vi "Convert filetype to Is VI.vi"(4 "file type":T1) -> (1 "Is VI?":bool)   [LabVIEW 2019, in "NI_FileType.lvlib"]
doc: "Returns TRUE if this file type could be loaded with the Open VI Reference function. It includes VIs, Polymorphic VIs, Controls, Templates, and Globals."
uses:
  NI_FileType.lvlib
  FT_FileTypes.ctl
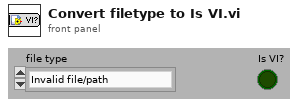
[diagram p1: front panel]
types:
  T1 = typedef "NI_FileType.lvlib/FT_FileTypes.ctl" = enum32{"Invalid file/path", "Unknown type", "Instrument", "Control", "Polymorphic VI", "Project", "Library", "LVClass", "XControl", "XNode", "CIN", "Run-time menu", "Palette menu", "LLB", "Shortcut", "Directory", "Class Private Data Control", "Statechart", "MathScript .m file", "Ladder Diagram", "LVLibp"}
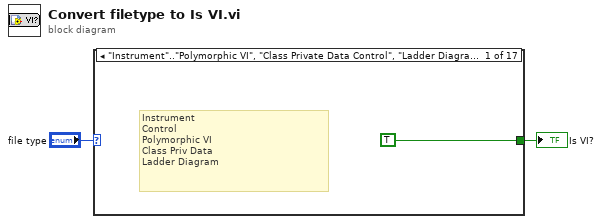
[diagram p0: block diagram]
diagram:
  n1 = case shown="\"Instrument\"..\"Polymorphic VI\", \"Class Private Data Control\", \"Ladder Diagram\"" "file type" {
    tunnel: [TRUE _ _ _ _ _ _ _ _ _ _ _ _ _ _ _ _] -> w2
    frame "Instrument".."Polymorphic VI", "Class Private Data Control", "Ladder Diagram" {
      # "Instrument\nControl\nPolymorphic VI\nClass Priv Data\nLadder Diagram"
    }
    frame "Project" {
    }
    frame "Library" {
    }
    frame "LVClass" {
    }
    frame "XControl" {
    }
    frame "XNode" {
    }
    frame "CIN" {
    }
    frame "Run-time menu" {
    }
    frame "Palette menu" {
    }
    frame "LLB" {
    }
    frame "Shortcut" {
    }
    frame "Directory" {
    }
    frame "Unknown type" {
    }
    frame "Invalid file/path" {
    }
    frame "Statechart" {
    }
    frame "MathScript .m file" {
    }
    frame "LVLibp" {
    }
  }
  "Is VI?" <- w2
